vi "fgv-locker.vi"() -> (1 "create new?":bool, 2 "Queue out":refnum<queue>)   [LabVIEW 2017, in "ObjectCacherAPI.lvlib"]
uses:
  ObjectCacherAPI.lvlib
  96c80c41-8aa5-4c9c-bf90-f049b60024d1.vi
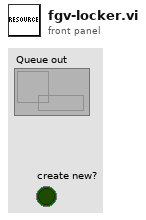
[diagram p1: front panel]
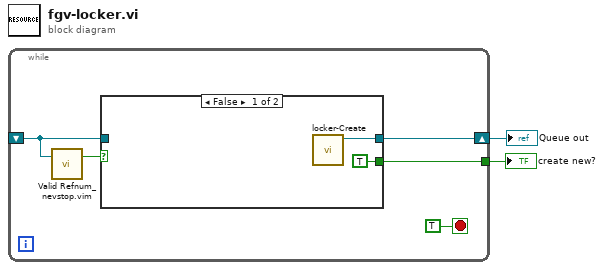
[diagram p0: block diagram]
diagram:
  n1 = while {
    shift-right: [w4] -> w2
    shift-left: _ -> [w5]
    tunnel: [w3] -> w1
    stop <- TRUE stop-if-true
    n2 = call "Valid Refnum_nevstop.vim"("number/path/refnum"=w5) -> ("Valid Number/Path/Refnum"=w6:bool)  [unwired: 2 in]
    n3 = case shown="False" w6 {
      tunnel: [w9 w10] -> w4
      tunnel: w5 -> [_ w10]
      tunnel: [TRUE _] -> w3
      frame False {
        n4 = call "locker-Create.vi"() -> ("Queue out"=w9:refnum<queue>)  [unwired: 10 in, 1 out]
      }
      frame True {
      }
    }
  }
  "Queue out" <- w2
  "create new?" <- w1
